vi "provide_note_book_info.vi"(8 "error in (no error)":errorcluster, 10 "notebook string in":string, 11 "StimulatorDL090727DAQmx in":refnum<class "StimulatorDL090727Writer.lvclass">) -> (0 "error out":errorcluster, 2 "notebook string out":string, 3 "StimulatorDL090727DAQmx out":refnum<class "StimulatorDL090727Writer.lvclass">)   [LabVIEW 2010, in "StimulatorDL090727Writer.lvclass"]
uses:
  StimulatorDL090727Writer.lvclass
  StimulatorDL090727Writer.lvclass/StimulatorDL090727Writer.ctl
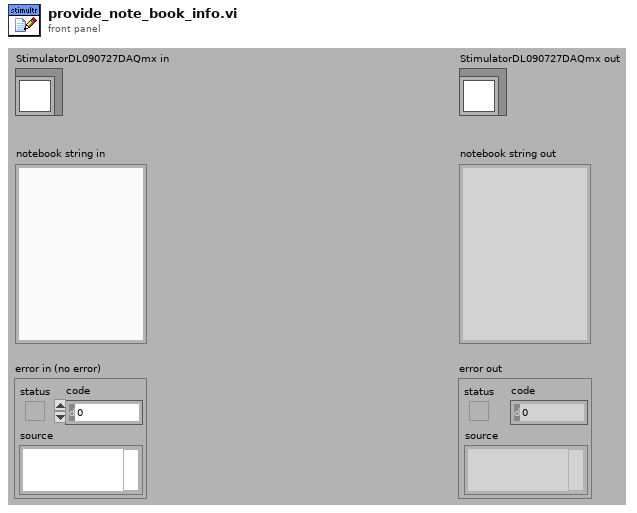
[diagram p1: front panel]
types:
  T1 = typedef "StimulatorDL090727Writer.lvclass/pattern_enum.ctl" = enum16{"sine wave", "square"}
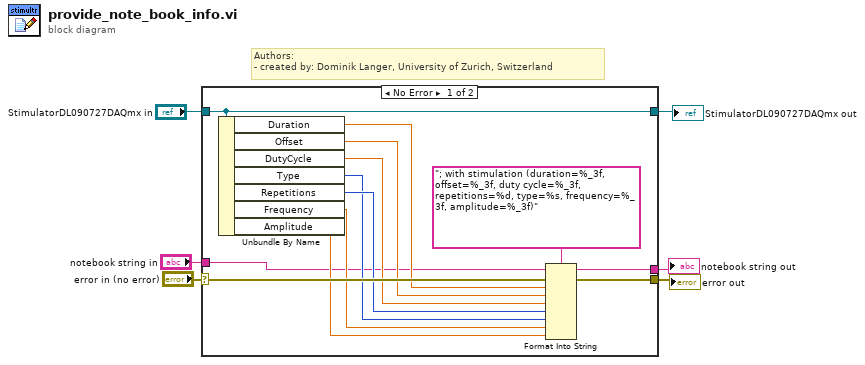
[diagram p0: block diagram]
diagram:
  # "Authors: \n- created by: Dominik Langer, University of Zurich, Switzerland"
  n1 = case shown="No Error" "error in (no error)" {
    selector: "error in (no error)" -> [w19 w22]
    tunnel: "StimulatorDL090727DAQmx in" -> [w18 w21]
    tunnel: [w17 w22] -> w4
    tunnel: [w18 w21] -> w3
    tunnel: "notebook string in" -> [w7 w20]
    tunnel: [w8 w20] -> w1
    frame No Error {
      n2 = Unbundle By Name(w18) -> ("Duration"=w15:dbl[unit], "Offset"=w14:dbl[unit], "DutyCycle"=w13:dbl[unit], "Type"=w11:T1, "Repetitions"=w12:i32, "Frequency"=w10:dbl[unit], "Amplitude"=w9:dbl)
      n3 = Format Into String(format string="; with stimulation (duration=%_3f, offset=%_3f, duty cycle=%_3f, repetitions=%d, type=%s, frequency=%_3f, amplitude=%_3f)" ("string"), initial string=w7, error in=w19, w15, w14, w13, w12, w11, w10, w9) -> (resulting string=w8:string, error out=w17:errorcluster)
    }
    frame Error {
    }
  }
  "error out" <- w4
  "StimulatorDL090727DAQmx out" <- w3
  "notebook string out" <- w1
